vi "EventBallAtGoalkeeperArea.vi"(9 "Field defense":dbl[](array[numeric]), 10 "IA State":T1={"our_robots"=[], "enemy_robots"=[], "balls"=[], "geometry"={"line_width"=0, "field_length"=0, "field_width"=0, "boundary_width"=0, "referee_width"=0, "goal_width"=0, "goal_depth"=0, "goal_wall_width"=0, "center_circle_radius"=0, "defense_radius"=0, "defense_stretch"=0, "free_kick_from_defense_dist"=0, "penalty_spot_from_field_line_dist"=0, "penalty_line_from_spot_dist"=0}, "IA Judge"={"stage"="", "command"="", "our_goalie_id"=0.0, "enemy_goalie_id"=0.0, "command enum"=enum."Halt", "Time"=enum."Azul"}, "Received Timestamp"=timestamp(0 s since 1904-01-01), "Events"={"Touch"=FALSE, "Ball out"=FALSE, "id touch"=0.0, "Ball out of \nVision"=FALSE, "Ball inside \nGoalie area"=FALSE, "Robot not responding"=FALSE, "Robots responding status"=[1.0, 1.0, 1.0, 1.0, 1.0, 1.0], "Enemy Ball \nPossession"=FALSE, "Pass State"=FALSE, "id end of pass"=0.0, "Kick"=FALSE, "Id ini Possession"=0.0, "Ball Possesion"=FALSE, "Id Possesion"=0.0}}) -> (2 "Ball at goalkeeper area ?":bool)   [LabVIEW 2017]
uses:
  Core/AI Input.ctl
  Core/AI Robot.ctl
  Intel/Functions Enum.ctl
  Intel/AttackerStates.ctl
  Path Planning/RRT/PathDests.ctl
  Path Planning/RRT/PathDest.ctl
  Core/AI Ball.ctl
  Core/Field Size.ctl
  Core/AI Judge.ctl
  Intel/Command Enum.ctl
  Events.ctl
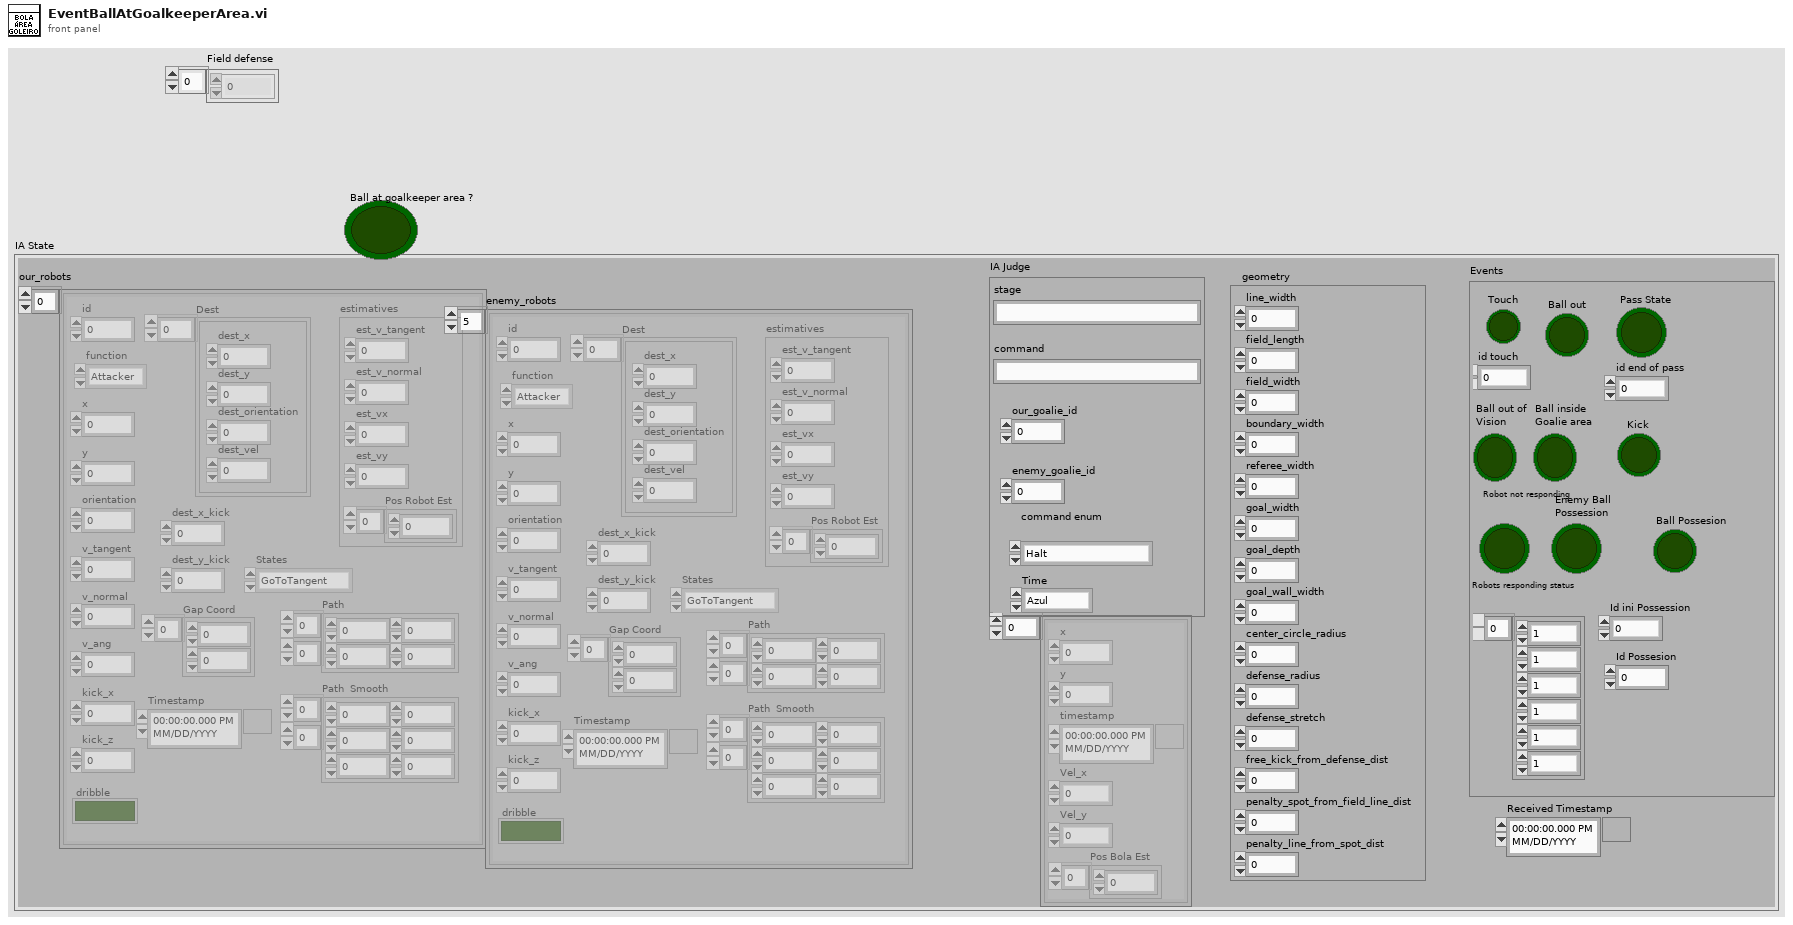
[diagram p1: front panel]
types:
  T1 = typedef "AI Input.ctl" = cluster{"our_robots":T2[], "enemy_robots":T2[], "balls":T7[], "geometry":T8, "IA Judge":T9, "Received Timestamp":timestamp, "Events":T11}
  T2 = typedef "AI Robot.ctl" = cluster{"id":u32, "function":T3, "x":dbl, "y":dbl, "orientation":dbl, "v_tangent":dbl, "v_normal":dbl, "v_ang":dbl, "kick_x":dbl, "kick_z":dbl, "dribble":bool, "Timestamp":timestamp, "estimatives":cluster{"est_v_tangent":dbl, "est_v_normal":dbl, "est_vx":dbl, "est_vy":dbl, "Pos Robot Est":dbl[]}, "dest_x_kick":dbl, "dest_y_kick":dbl, "Gap Coord":dbl[], "States":T4, "Path ":dbl[][], "Path  Smooth":dbl[][], "Dest":T5}
  T3 = typedef "Functions Enum.ctl" = enum16{"Attacker", "Goalie", "Defender", "Striker", "Goto 0", "Dummy", "Kicker", "ZigZag 0", "ZigZag 1", "ZigZag 2", "ZigZag 3", "ZigZag 4", "ZigZag 5", "ZigZag 6", "ZigZag 7", "ZigZag 8", ""}
  T4 = typedef "AttackerStates.ctl" = enum16{"Pass", "GoToTangent", "BallGetting", "GoToKick", ""}
  T5 = typedef "PathDests.ctl" = T6[]
  T6 = typedef "PathDest.ctl" = cluster{"dest_x":dbl, "dest_y":dbl, "dest_orientation":dbl, "dest_vel":dbl}
  T7 = typedef "AI Ball.ctl" = cluster{"x":dbl, "y":dbl, "timestamp":timestamp, "Vel_x":dbl, "Vel_y":dbl, "Pos Bola Est":dbl[]}
  T8 = typedef "Field Size.ctl" = cluster{"line_width":u32, "field_length":u32, "field_width":u32, "boundary_width":u32, "referee_width":u32, "goal_width":u32, "goal_depth":u32, "goal_wall_width":u32, "center_circle_radius":u32, "defense_radius":u32, "defense_stretch":u32, "free_kick_from_defense_dist":u32, "penalty_spot_from_field_line_dist":u32, "penalty_line_from_spot_dist":u32}
  T9 = typedef "AI Judge.ctl" = cluster{"stage":string, "command":string, "our_goalie_id":dbl, "enemy_goalie_id":dbl, "command enum":T10, "Time":enum16{"Azul", "Amarelo"}}
  T10 = typedef "Command Enum.ctl" = enum16{"Halt", "Stop", "Force Start", "PKA Normal Start", "Prepare Kickoff Ally", "PKE Normal Start", "Prepare Kickoff Enemy", "Prepare Penalty Ally", "PPA Normal Start", "Prepare Penalty Enemy", "PPE Normal Start", "Direct Free Enemy", "Direct Free Ally", "Indirect Free Enemy", "Indirect Free Ally", "Timeout Enemy", "Timeout Ally", "Goal Enemy", "Goal Ally", "Ball Placement Enemy", "Ball Placement Ally", "Normal Half Time", "Extra Time Break", "Extra Half Time", "None", "Post Game"}
  T11 = typedef "Events.ctl" = cluster{"Touch":bool, "Ball out":bool, "id touch":dbl, "Ball out of \nVision":bool, "Ball inside \nGoalie area":bool, "Robot not responding":bool, "Robots responding status":dbl[], "Enemy Ball \nPossession":bool, "Pass State":bool, "id end of pass":dbl, "Kick":bool, "Id ini Possession":dbl, "Ball Possesion":bool, "Id Possesion":dbl}
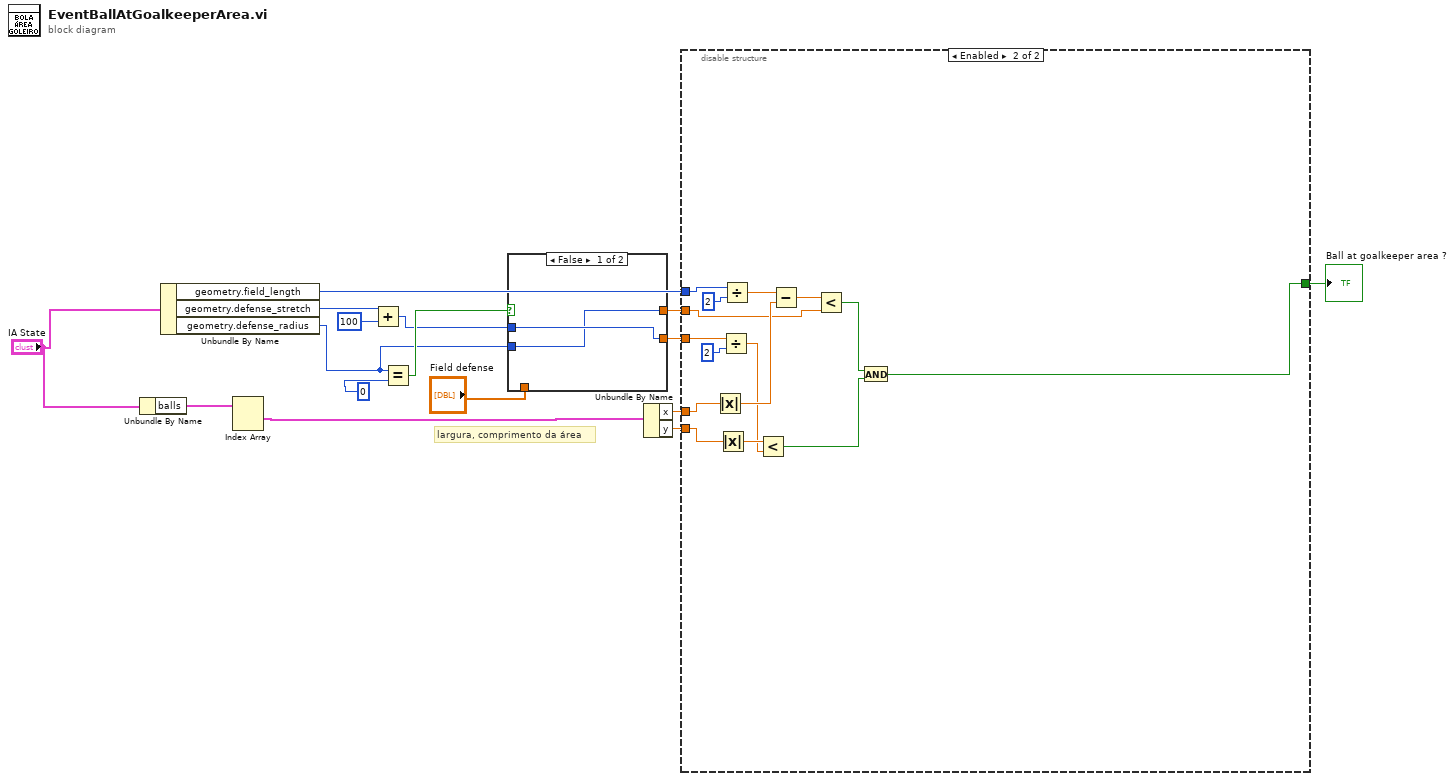
[diagram p0: block diagram]
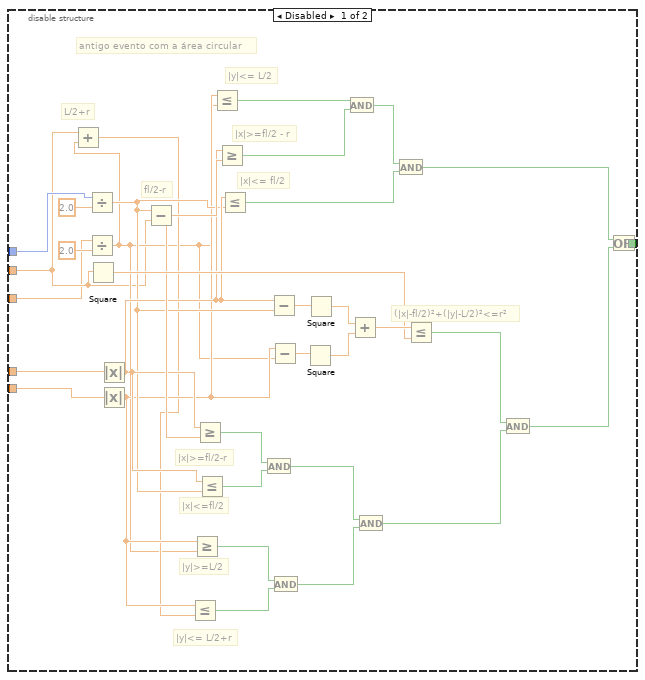
[diagram p2: hidden frame]
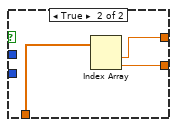
[diagram p3: hidden frame]
diagram:
  # "largura, comprimento da área"
  n1 = Unbundle By Name("IA State") -> ("balls"=w16:T7[])
  n2 = Unbundle By Name("IA State") -> ("geometry.field_length"=w12:u32, "geometry.defense_stretch"=w3:u32, "geometry.defense_radius"=w5:u32)
  n3 = Index Array(array=w16) -> (element #1=w4:T7)  [unwired: 2 in, 1 out]
  n4 = Add(x=w3, y=u32 100) -> (x+y=w2:u32)
  n5 = Equal?(x=w5, y=u32 0) -> (x = y?=w8:bool)
  n6 = case shown="False" w8 {
    tunnel: [w17 w21] -> w7
    tunnel: [w18 w20] -> w6
    tunnel: "Field defense" -> [_ w19]
    tunnel: w2 -> [w18 _]
    tunnel: w5 -> [w17 _]
    frame False {
    }
    frame True {
      n7 = Index Array(array=w19) -> (element #1=w21:dbl, element #2=w20:dbl)  [unwired: 2 in]
    }
  }
  n8 = Unbundle By Name(w4) -> ("x"=w13:dbl, "y"=w14:dbl)
  n9 = disable-structure shown="Enabled" {
    disable-tunnel: w14 -> [w55 w69]
    disable-tunnel: w13 -> [w54 w70]
    disable-tunnel: w12 -> [w51 w68]
    disable-tunnel: [w25 w56] -> w11
    disable-tunnel: w7 -> [w23 w62]
    disable-tunnel: w6 -> [w22 w60]
    frame Disabled {
      # "antigo evento com a área circular"
      # "|y|<= L/2+r"
      # "L/2+r"
      # "|y|>=L/2"
      # "|x|<=fl/2"
      # "|x|>=fl/2-r"
      # "fl/2-r"
      # "(|x|-fl/2)²+(|y|-L/2)²<=r²"
      # "|x|<= fl/2"
      # "|x|>=fl/2 - r"
      # "|y|<= L/2"
      n10 = Divide(x=w51, y=2.0) -> (x/y=w36:dbl)
      n11 = Divide(x=w22, y=2.0) -> (x/y=w24:dbl)
      n12 = Add(x=w23, y=w24) -> (x+y=w34:dbl)
      n13 = Square(x=w23) -> (x^2=w41:dbl)
      n14 = Absolute Value(x=w54) -> (abs(x)=w39:dbl)
      n15 = Absolute Value(x=w55) -> (abs(x)=w35:dbl)
      n16 = Subtract(x=w36, y=w23) -> (x-y=w40:dbl)
      n17 = Less Or Equal?(x=w35, y=w34) -> (x <= y?=w32:bool)
      n18 = Greater Or Equal?(x=w35, y=w24) -> (x >= y?=w33:bool)
      n19 = Greater Or Equal?(x=w39, y=w40) -> (x >= y?=w38:bool)
      n20 = Less Or Equal?(x=w39, y=w36) -> (x <= y?=w37:bool)
      n21 = Less Or Equal?(x=w35, y=w24) -> (x <= y?=w50:bool)
      n22 = Greater Or Equal?(x=w39, y=w40) -> (x >= y?=w49:bool)
      n23 = Less Or Equal?(x=w39, y=w36) -> (x <= y?=w47:bool)
      n24 = And(x=w38, y=w37) -> (x .and. y?=w31:bool)
      n25 = Subtract(x=w39, y=w36) -> (x-y=w46:dbl)
      n26 = Subtract(x=w35, y=w24) -> (x-y=w45:dbl)
      n27 = And(x=w33, y=w32) -> (x .and. y?=w30:bool)
      n28 = Square(x=w45) -> (x^2=w43:dbl)
      n29 = Square(x=w46) -> (x^2=w44:dbl)
      n30 = And(x=w50, y=w49) -> (x .and. y?=w48:bool)
      n31 = Add(x=w44, y=w43) -> (x+y=w42:dbl)
      n32 = And(x=w31, y=w30) -> (x .and. y?=w28:bool)
      n33 = And(x=w48, y=w47) -> (x .and. y?=w27:bool)
      n34 = Less Or Equal?(x=w42, y=w41) -> (x <= y?=w29:bool)
      n35 = And(x=w29, y=w28) -> (x .and. y?=w26:bool)
      n36 = Or(x=w27, y=w26) -> (x .or. y?=w25:bool)
    }
    frame Enabled {
      n37 = Absolute Value(x=w70) -> (abs(x)=w64:dbl)
      n38 = Absolute Value(x=w69) -> (abs(x)=w66:dbl)
      n39 = Divide(x=w60, y=u32 2) -> (x/y=w59:dbl)
      n40 = Divide(x=w68, y=u32 2) -> (x/y=w65:dbl)
      n41 = Less?(x=w66, y=w59) -> (x < y?=w57:bool)
      n42 = Subtract(x=w65, y=w64) -> (x-y=w63:dbl)
      n43 = Less?(x=w63, y=w62) -> (x < y?=w58:bool)
      n44 = And(x=w58, y=w57) -> (x .and. y?=w56:bool)
    }
  }
  "Ball at goalkeeper area ?" <- w11
